vi "sum.vi"() -> (3 "x+y":dbl)   [LabVIEW 2023]
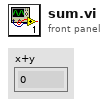
[diagram p1: front panel]
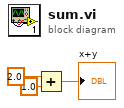
[diagram p0: block diagram]
diagram:
  n1 = Add(x=2.0, y=1.0) -> (x+y=→"x+y":dbl)
